vi "move speed.vi"(0 "X":dbl, 7 "i":i32, 9 "speed":dbl, 11 "dt(s)":dbl, 12 "t3 in":dbl) -> (2 "t2":dbl, 6 "speed out":dbl, 10 "t2?":bool, 14 "t3":dbl, 15 "complet?":bool)   [LabVIEW 2019]
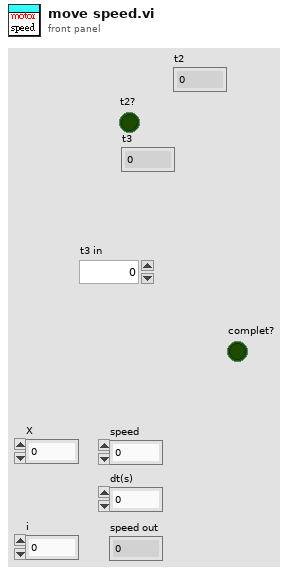
[diagram p1: front panel]
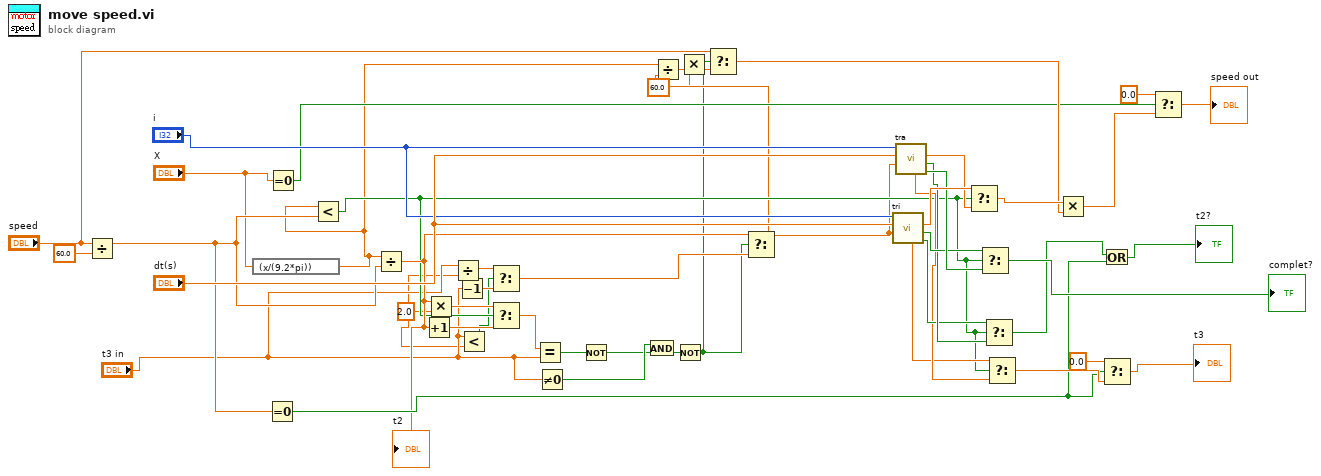
[diagram p0: block diagram]
diagram:
  w4 = 2.0 ("y")
  n1 = Divide(x="speed", y=60.0) -> (x/y=w31:dbl)
  n2 = expression code="(x/(9.2*pi))"("X") -> (w13:dbl)
  n3 = Equal To 0?(x=w31) -> (x = 0?=w32:bool)
  n4 = Equal To 0?(x="X") -> (x = 0?=w14:bool)
  n5 = Less?(x=w13, y=w31) -> (x < y?=w20:bool)
  n6 = Divide(x=w13, y=w31) -> (x/y=w22:dbl)
  "t2" <- w22
  n7 = Increment(x=w22) -> (x+1=w24:dbl)
  n8 = Multiply(x=w22, y=w4) -> (x*y=w21:dbl)
  n9 = Divide(x="t3 in", y=w4) -> (x/y=w19:dbl)
  n10 = Decrement(x="t3 in") -> (x-1=w18:dbl)
  n11 = Less?(x="t3 in", y=w4) -> (x < y?=w3:bool)
  n12 = Select(t=w19, s=w3, f=w18) -> (s? t:f=w17:dbl)
  n13 = Select(t=w21, s=w20, f=w24) -> (s? t:f=w23:dbl)
  n14 = Equal?(x=w23, y="t3 in") -> (x = y?=w10:bool)
  n15 = Not Equal To 0?(x="t3 in") -> (x != 0?=w8:bool)
  n16 = Not(x=w10) -> (.not. x?=w7:bool)
  n17 = And(x=w8, y=w7) -> (x .and. y?=w9:bool)
  n18 = Not(x=w9) -> (.not. x?=w6:bool)
  n19 = Select(t=w22, s=w6, f=w17) -> (s? t:f=w12:dbl)
  n20 = Divide(x=w13, y=w12) -> (x/y=w11:dbl)
  n21 = Multiply(x=60.0, y=w11) -> (x*y=w2:dbl)
  n22 = Select(t="speed", s=w6, f=w2) -> (s? t:f=w16:dbl)
  n23 = call "tri.vi"("t2"=w12, "dt(s)"="dt(s)", "i"="i") -> ("t2?"=w39:bool, "complet?"=w43:bool, "Waveform Chart"=w46:dbl, "t3"=w25:dbl)  [unwired: 5 in]
  n24 = call "tra.vi"("t2"=w12, "dt(s)"="dt(s)", "i"="i") -> ("complet?"=w44:bool, "t2?"=w40:bool, "Waveform Chart"=w45:dbl, "t3"=w38:dbl)  [unwired: 4 in, 1 out]
  n25 = Select(t=w46, s=w20, f=w45) -> (s? t:f=w41:dbl)
  n26 = Select(t=w43, s=w20, f=w44) -> (s? t:f=→"complet?":bool)
  n27 = Select(t=w39, s=w20, f=w40) -> (s? t:f=w34:bool)
  n28 = Select(t=w25, s=w20, f=w38) -> (s? t:f=w36:dbl)
  n29 = Multiply(x=w41, y=w16) -> (x*y=w27:dbl)
  n30 = Or(x=w34, y=w32) -> (x .or. y?=→"t2?":bool)
  n31 = Select(t=0.0, s=w32, f=w36) -> (s? t:f=→"t3":dbl)
  n32 = Select(t=0.0, s=w14, f=w27) -> (s? t:f=→"speed out":dbl)
